vi "Main.vi"() -> ()   [LabVIEW 2024]
doc: "This template is for the Queued Message Handler design pattern.\n\nThe Event Handling Loop generates messages based on user interface actions.\n\nThe Message Handling Loop processes messages generated by the Event Handling Loop, or by other messages. The messages are string values, so new messages can be added easily to the Message Cases case structure in the Message Handling Loop. Each message cluster can also provide an optional value for Message Data, which is a variant that can be converted to whatever message-specific data is required."
uses:
  support/Message Queue/Enqueue Message (Single).vi
  <vilib>/Utility/error.llb/Error Cluster From Error Code.vi
  <vilib>/ErrorRing/Error Ring.xnode
  support/Message Queue/Message Queue.lvlib
  support/User Event - Stop/User Event - Stop.lvlib
panel:
  in  "Path":path
  out "Waveform Graph":dbl[](graph)
  out "Status":string
  in  "Open file":bool
  in  "Exit":bool
  # "File Reader lab 5"
  # "C:\\Users\\danfr\\Documents\\Studie\\V25\\FYS4240 - Datainnsamling og Kontroll\\Lab\\lab5_v25\\Example Binary File.dat"
  # "Path to the binary file on my computer"
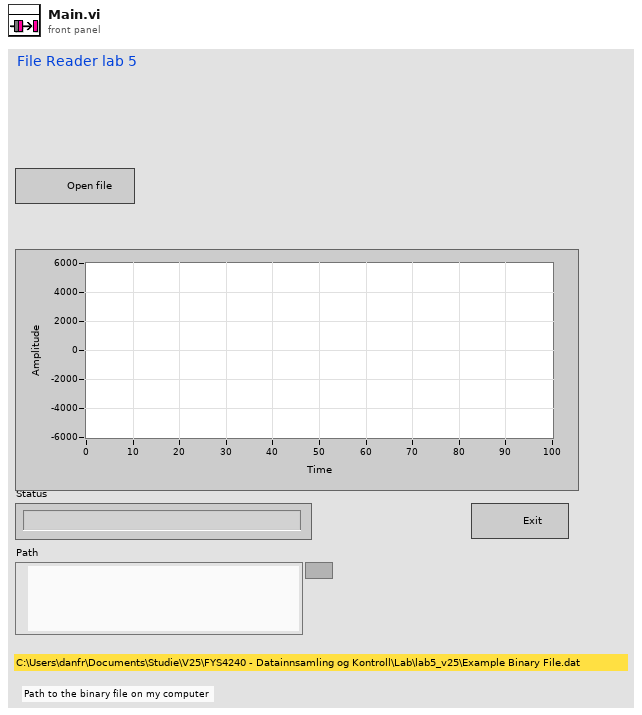
[diagram p1: front panel]
types:
  T1 = typedef "Message Queue.lvlib/All Message Queues.ctl" = cluster{"UI":refnum<queue>}
  T2 = enum16{"open", "replace", "create", "open or create", "replace or create", "replace or create with confirmation"}
  T3 = enum16{"big-endian, network order", "native, host order", "little-endian"}
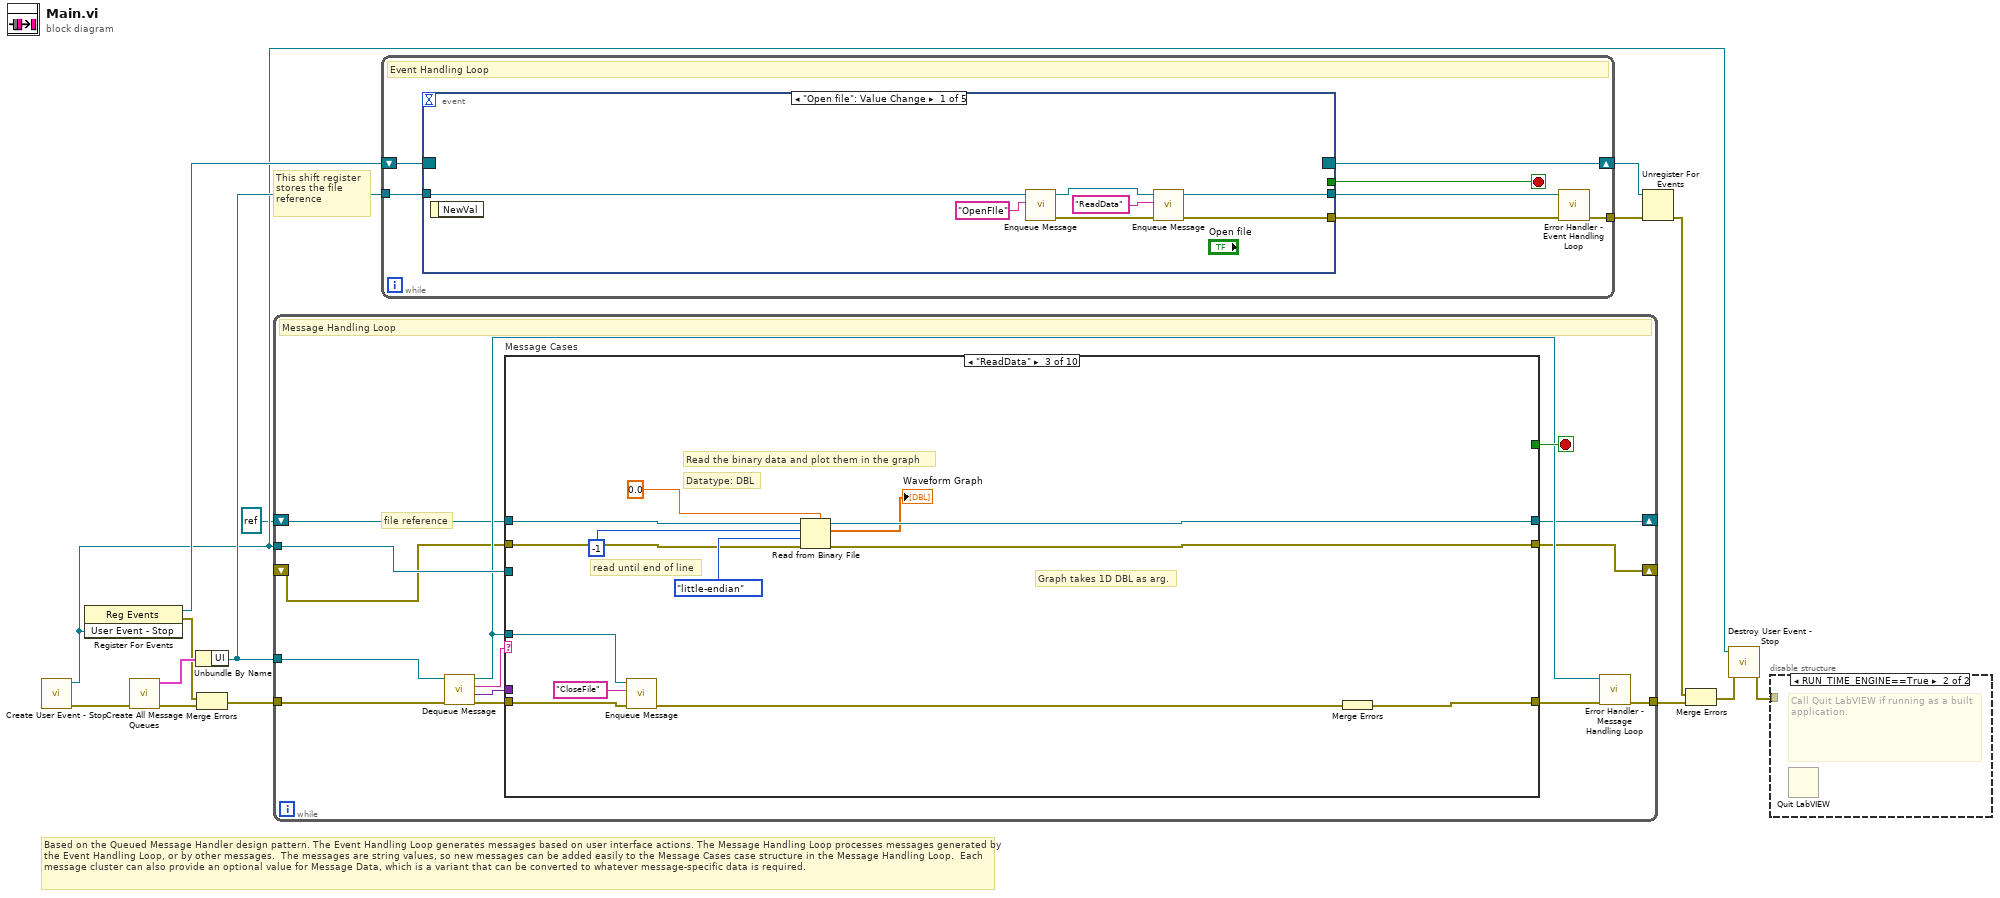
[diagram p0: block diagram]
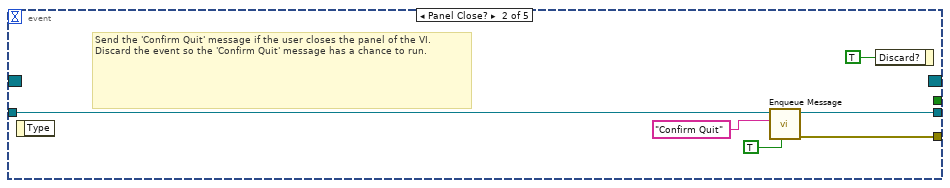
[diagram p3: hidden frame]
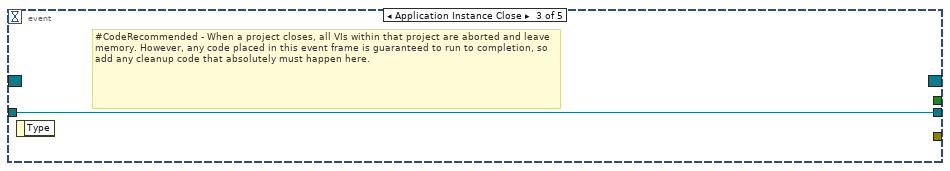
[diagram p4: hidden frame]
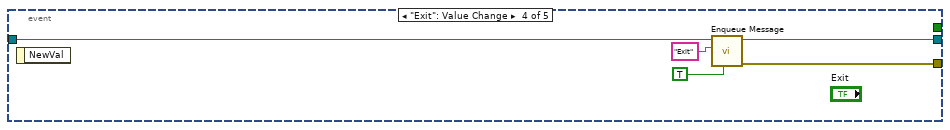
[diagram p5: hidden frame]
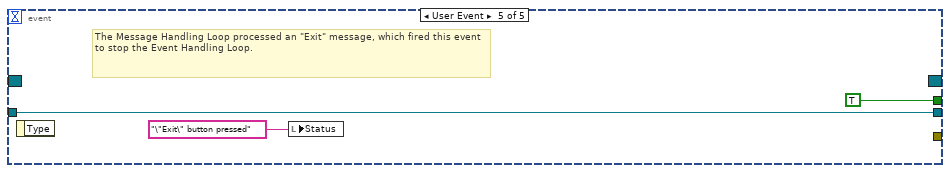
[diagram p6: hidden frame]
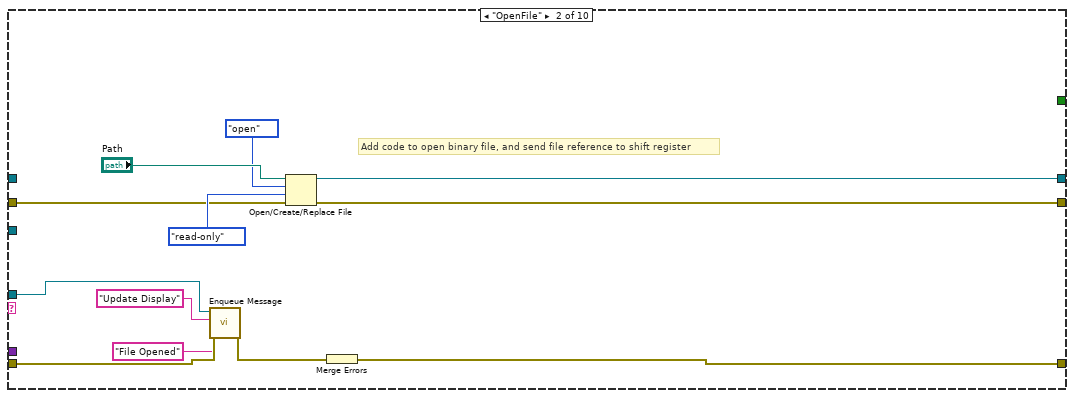
[diagram p8: hidden frame]
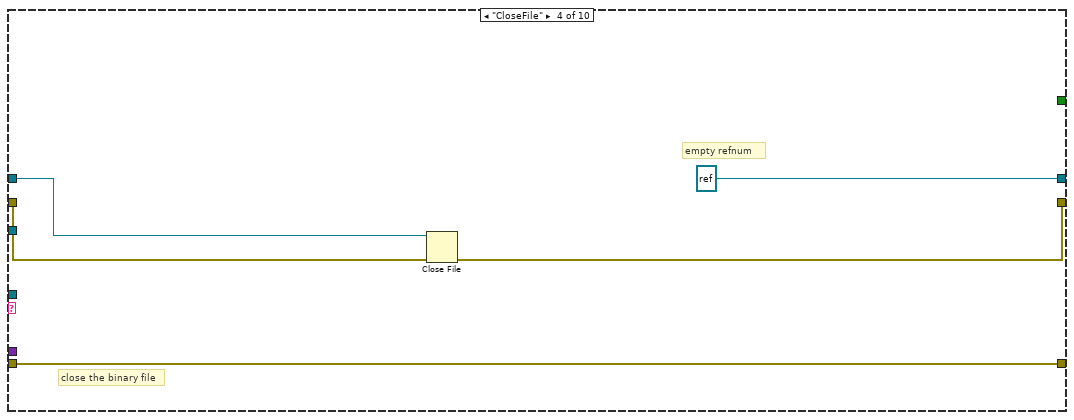
[diagram p9: hidden frame]
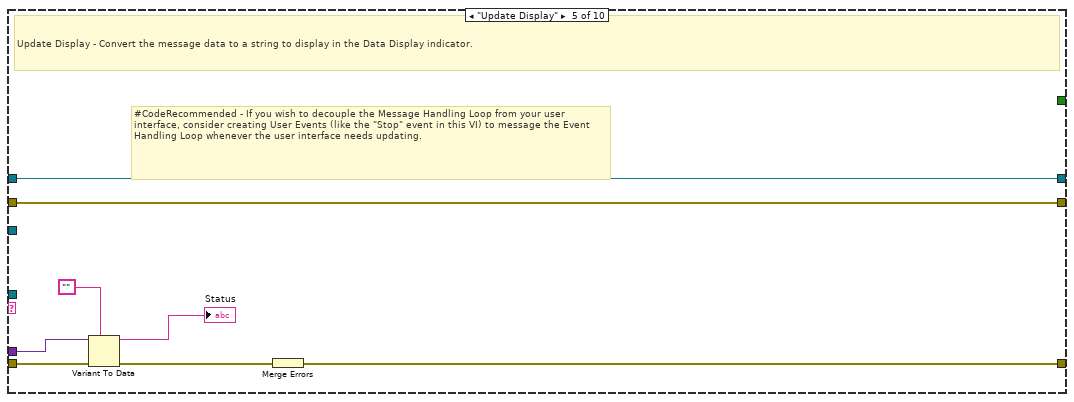
[diagram p10: hidden frame]
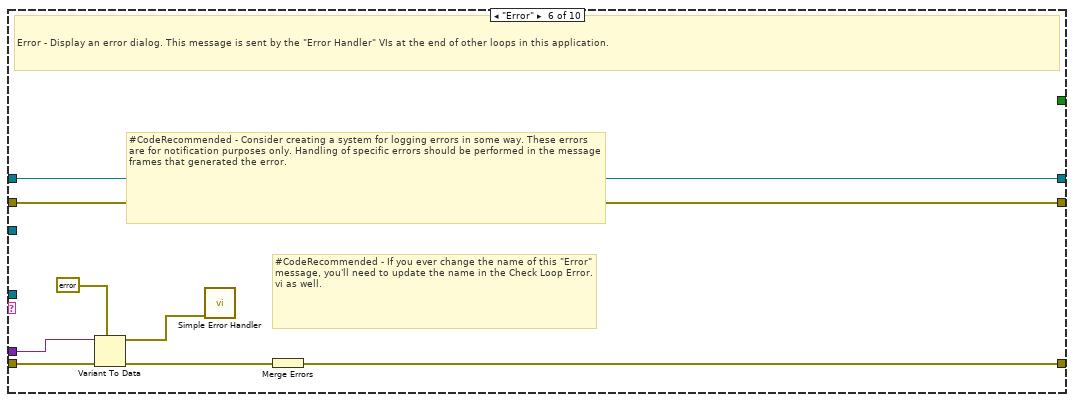
[diagram p11: hidden frame]
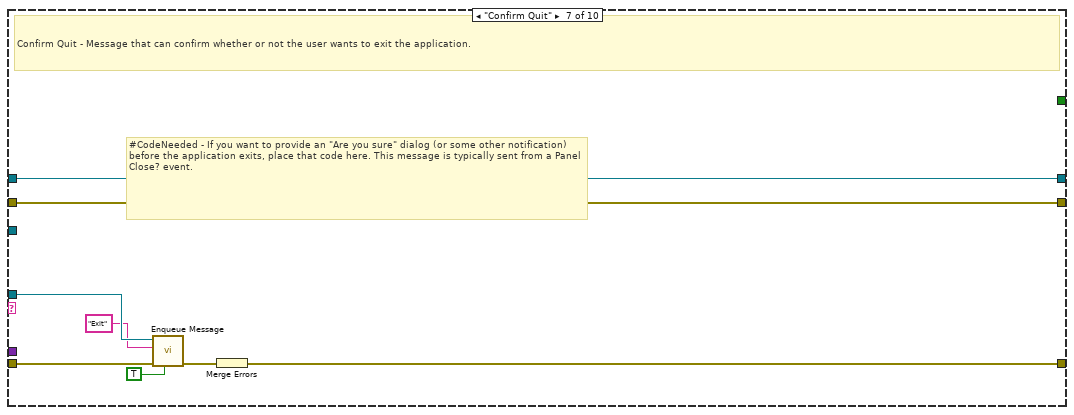
[diagram p12: hidden frame]
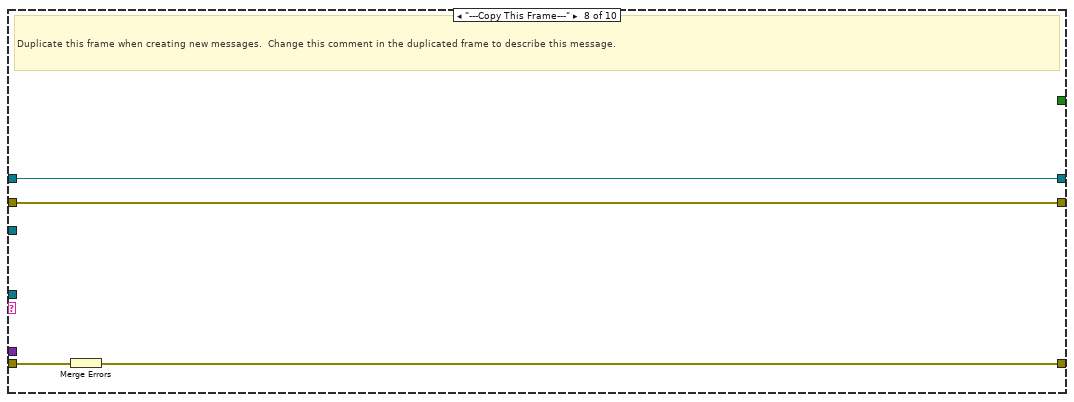
[diagram p13: hidden frame]
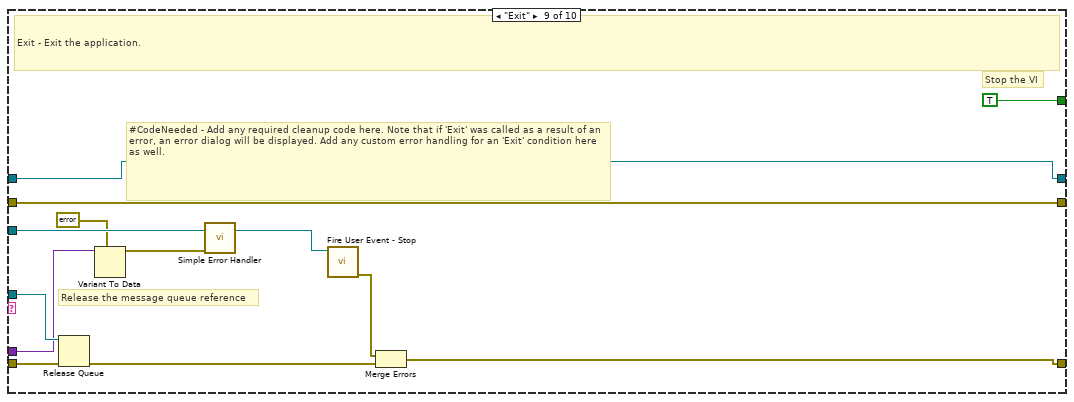
[diagram p14: hidden frame]
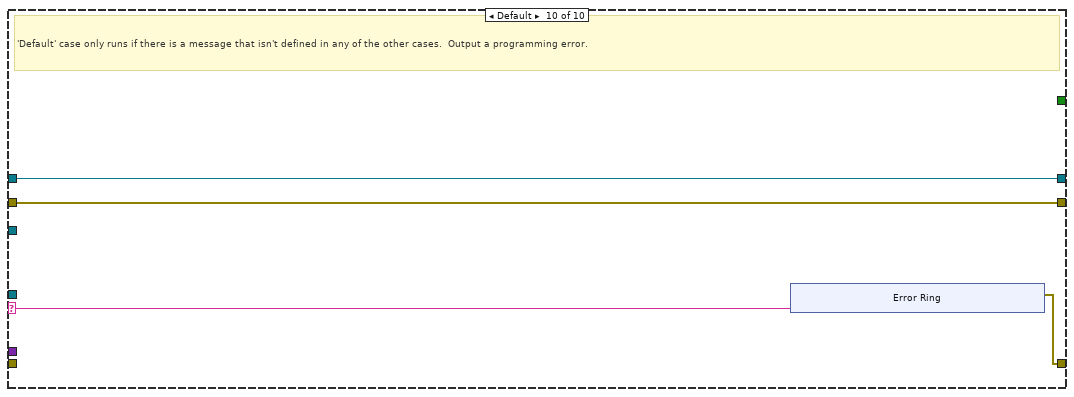
[diagram p15: hidden frame]
diagram:
  # "Based on the Queued Message Handler design pattern. The Event Handling Loop generates messages based on user interface actions. The Message Handling Loop processes messages generated by the Event Handling Loop, or by other messages.  The messages are string values, so new messages can be added easily to the Message Cases case structure in the Message Handling Loop.  Each message cluster can also provide an optional value for Message Data, which is a variant that can be converted to whatever message-specific data is required."
  # "This shift register stores the file reference"
  n1 = call "Create User Event - Stop.vi"() -> ("error out"=w11:errorcluster, "User Event - Stop"=w4:refnum<user-event>)  [unwired: 10 in]
  n2 = register-events(w4) -> (reference out=w5:refnum<event-registration>, error out=w2:errorcluster)  [unwired: 2 in]
  n3 = call "Create All Message Queues.vi"("error in (no error)"=w11) -> ("error out"=w15:errorcluster, "Message Queues out"=w14:T1)  [unwired: 9 in]
  n4 = Unbundle By Name(w14) -> ("UI"=w12:refnum<queue>)
  n5 = Merge Errors(w2, w15) -> (w3:errorcluster)
  n6 = while {
    tunnel: w12 -> [w23]
    tunnel: w4 -> [w28]
    tunnel: w3 -> [w27]
    tunnel: [w21] -> w13
    shift-right: [w18] -> _
    shift-left: refnum<file> refnum ("refnum out") -> [w19]
    shift-right: [w17] -> _
    shift-left: _ -> [w16]
    stop <- w29 stop-if-true
    # "file reference"
    # "Message Handling Loop"
    n7 = call "Dequeue Message.vi"("error in (no error)"=w27, "Message Queue"=w23) -> ("error out"=w26:errorcluster, "Message Data"=w24:variant, "Message"=w25:string, "dup Message Queue"=w22:refnum<queue>)  [unwired: 6 in]
    n8 = case "Message Cases" shown="\"ReadData\"" w25 {
      selector: w25 -> [_ _ _ _ _ _ _ _ _ w105]
      tunnel: w22 -> [_ w41 w54 _ _ _ w83 _ w102 _]
      tunnel: w26 -> [w32 w43 w56 w62 w69 w78 w86 w90 w96 _]
      tunnel: [w32 w44 w57 w62 w70 w73 w85 w89 w99 w106] -> w20
      tunnel: [_ _ _ _ _ _ _ _ TRUE _] -> w29
      tunnel: w24 -> [_ _ _ _ w68 w77 _ _ w93 _]
      tunnel: w28 -> [_ _ _ _ _ _ _ _ w98 _]
      tunnel: w19 -> [w31 _ w52 w61 w64 w72 w80 w88 w92 w104]
      tunnel: [w31 w36 w51 refnum<file> refnum ("refnum") w64 w72 w80 w88 w92 w104] -> w18
      tunnel: [w30 w33 w46 w59 w63 w71 w79 w87 w91 w103] -> w17
      tunnel: w16 -> [w30 w34 w45 w58 w63 w71 w79 w87 w91 w103]
      frame "Initialize" {
        # "Nothing added here in this example"
        # "Initialize - All initialization work should take place in this message, since other loops can potentially enqueue messages that execute immediately after this one."
      }
      frame "OpenFile" {
        # "Add code to open binary file, and send file reference to shift register"
        n9 = call-poly "Enqueue Message.vi"("error in (no error)"=w43, "Message Data"="File Opened" ("\"Do Something\" button pressed"), "Message"="Update Display", "Message Queue"=w41) -> ("error out"=w42:errorcluster)  [unwired: 6 in, 1 out]
        n10 = Open/Create/Replace File(file path (use dialog)="Path", error in=w34, operation (0:open)=T2."open", access (0:read/write)=enum16{"read/write", "read-only", "write-only"}."read-only") -> (refnum out=w36:refnum<file>, error out=w33:errorcluster)  [unwired: 2 in, 1 out]
        n11 = Merge Errors(w42) -> (w44:errorcluster)
      }
      frame "ReadData" {
        # "read until end of line"
        # "Graph takes 1D DBL as arg."
        # "Datatype: DBL"
        # "Read the binary data and plot them in the graph"
        n12 = call-poly "Enqueue Message.vi"("error in (no error)"=w56, "Message"="CloseFile", "Message Queue"=w54) -> ("error out"=w55:errorcluster)  [unwired: 7 in, 1 out]
        n13 = Read from Binary File(5:0.0, 8:w45, 9:T3."little-endian" ("byte order (0:big-endian, network order)"), 10:-1 ("count (1)"), 11:w52) -> (0:w46:errorcluster, 2:→"Waveform Graph":dbl[], 3:w51:refnum<file>)  [unwired: 1 in, 1 out]
        n14 = Merge Errors(w55) -> (w57:errorcluster)
      }
      frame "CloseFile" {
        # "empty refnum"
        # "close the binary file"
        n15 = Close File(refnum=w61, error in=w58) -> (error out=w59:errorcluster)  [unwired: 1 out]
      }
      frame "Update Display" {
        # "#CodeRecommended - If you wish to decouple the Message Handling Loop from your user interface, consider creating User Events (like the \"Stop\" event in this VI) to message the Event Handling Loop whenever the user interface needs updating."
        # "Update Display - Convert the message data to a string to display in the Data Display indicator."
        n16 = Variant To Data(error in=w69, type="", Variant=w68) -> (data=→"Status":string, error out=w66:errorcluster)
        n17 = Merge Errors(w66) -> (w70:errorcluster)
      }
      frame "Error" {
        # "#CodeRecommended - If you ever change the name of this \"Error\" message, you'll need to update the name in the Check Loop Error.vi as well."
        # "#CodeRecommended - Consider creating a system for logging errors in some way. These errors are for notification purposes only. Handling of specific errors should be performed in the message frames that generated the error."
        # "Error - Display an error dialog. This message is sent by the \"Error Handler\" VIs at the end of other loops in this application."
        n18 = Variant To Data(error in=w78, type=errorcluster {"status"=FALSE, "code"=0, "source"=""} ("error constant"), Variant=w77) -> (data=w75:errorcluster, error out=w74:errorcluster)
        n19 = call <vilib>:"Simple Error Handler.vi"("error in (no error)"=w75) -> ()  [unwired: 4 in, 5 out]
        n20 = Merge Errors(w74) -> (w73:errorcluster)
      }
      frame "Confirm Quit" {
        # "#CodeNeeded - If you want to provide an \"Are you sure\" dialog (or some other notification) before the application exits, place that code here. This message is typically sent from a Panel Close? event."
        # "Confirm Quit - Message that can confirm whether or not the user wants to exit the application."
        n21 = call-poly "Enqueue Message.vi"("Priority Message? (F)"=TRUE, "error in (no error)"=w86, "Message"="Exit", "Message Queue"=w83) -> ("error out"=w84:errorcluster)  [unwired: 6 in, 1 out]
        n22 = Merge Errors(w84) -> (w85:errorcluster)
      }
      frame "---Copy This Frame---" {
        # "Duplicate this frame when creating new messages.  Change this comment in the duplicated frame to describe this message."
        n23 = Merge Errors(w90) -> (w89:errorcluster)
      }
      frame "Exit" {
        # "Stop the VI"
        # "Release the message queue reference"
        # "#CodeNeeded - Add any required cleanup code here. Note that if 'Exit' was called as a result of an error, an error dialog will be displayed. Add any custom error handling for an 'Exit' condition here as well."
        # "Exit - Exit the application."
        n24 = Release Queue(queue=w102, error in (no error)=w96) -> (error out=w100:errorcluster)  [unwired: 1 in, 2 out]
        n25 = Variant To Data(type=errorcluster {"status"=FALSE, "code"=0, "source"=""} ("error constant"), Variant=w93) -> (data=w94:errorcluster)  [unwired: 1 in, 1 out]
        n26 = call <vilib>:"Simple Error Handler.vi"("error in (no error)"=w94) -> ()  [unwired: 4 in, 5 out]
        n27 = call "Fire User Event - Stop.vi"("User Event - Stop"=w98) -> ("error out"=w97:errorcluster)  [unwired: 10 in]
        n28 = Merge Errors(w97, w100) -> (w99:errorcluster)
      }
      frame Default {
        # "'Default' case only runs if there is a message that isn't defined in any of the other cases.  Output a programming error."
        n29 = xnode "Error Ring"("parameter 0"=w105) -> ("error out"=w106:errorcluster)
      }
    }
    n30 = call "Error Handler - Message Handling Loop.vi"("error in (no error)"=w20, "Message Queue"=w22) -> ("dup error in"=w21:errorcluster)  [unwired: 8 in, 1 out]
  }
  n31 = while {
    tunnel: w12 -> [w120]
    shift-right: [w118] -> w8
    shift-left: w5 -> [w119]
    tunnel: [w114] -> w6
    stop <- w116 stop-if-true
    # "Event Handling Loop"
    n32 = event shown="[0] \"Open file\": Value Change" {
      selector: w119 -> [_ _ _ _ _]
      dyn-events: [_ _ _ _ _] -> w118
      timeout: _ -> [_ _ _ _ _]
      tunnel: [_ _ _ _ TRUE ("Discard?")] -> w116
      tunnel: w120 -> [w127 w132 w134 w139 w142]
      tunnel: [w121 w131 _ w138 _] -> w117
      tunnel: [w122 w130 w134 w137 w142] -> w115
      event "Open file": Value Change {
        n33 = event-data() -> ()  [unwired: 1 in, 1 out]
        n34 = call-poly "Enqueue Message.vi"("Message"="OpenFIle", "Message Queue"=w127) -> ("error out"=w124:errorcluster, "dup Message Queue"=w125:refnum<queue>)  [unwired: 8 in]
        n35 = call-poly "Enqueue Message.vi"("error in (no error)"=w124, "Message"="ReadData", "Message Queue"=w125) -> ("error out"=w121:errorcluster, "dup Message Queue"=w122:refnum<queue>)  [unwired: 7 in]
      }
      event Panel Close? {
        # "Send the 'Confirm Quit' message if the user closes the panel of the VI. Discard the event so the 'Confirm Quit' message has a chance to run."
        n36 = event-data() -> ()  [unwired: 1 in, 1 out]
        n37 = call-poly "Enqueue Message.vi"("Priority Message? (F)"=TRUE, "Message"="Confirm Quit", "Message Queue"=w132) -> ("error out"=w131:errorcluster, "dup Message Queue"=w130:refnum<queue>)  [unwired: 7 in]
        n38 = event-data("Discard?"=TRUE) -> ()  [unwired: 1 in, 1 out]
      }
      event Application Instance Close {
        # "#CodeRecommended - When a project closes, all VIs within that project are aborted and leave memory. However, any code placed in this event frame is guaranteed to run to completion, so add any cleanup code that absolutely must happen here."
        n39 = event-data() -> ()  [unwired: 1 in, 1 out]
      }
      event "Exit": Value Change {
        n40 = event-data() -> ()  [unwired: 1 in, 1 out]
        n41 = call-poly "Enqueue Message.vi"("Priority Message? (F)"=TRUE, "Message"="Exit", "Message Queue"=w139) -> ("error out"=w138:errorcluster, "dup Message Queue"=w137:refnum<queue>)  [unwired: 7 in]
      }
      event User Event {
        # "The Message Handling Loop processed an \"Exit\" message, which fired this event to stop the Event Handling Loop."
        n42 = event-data() -> ()  [unwired: 1 in, 1 out]
        n43 = local write "Status"("\"Exit\" button pressed" ("VI Stopped")) -> ()
      }
    }
    n44 = call "Error Handler - Event Handling Loop.vi"("error in (no error)"=w117, "Message Queue"=w115) -> ("dup error in"=w114:errorcluster)  [unwired: 8 in, 1 out]
  }
  n45 = Unregister For Events(event registration refnum=w8, error in=w6) -> (error out=w9:errorcluster)
  n46 = Merge Errors(w9, w13) -> (w10:errorcluster)
  n47 = call "Destroy User Event - Stop.vi"("error in (no error)"=w10, "User Event - Stop"=w4) -> ("error out"=w7:errorcluster)  [unwired: 9 in]
  n48 = disable-structure shown="RUN_TIME_ENGINE==True" {
    disable-tunnel: w7 -> [_ _]
    frame condition #0 (active) {
    }
    frame condition #1 {
      # "Call Quit LabVIEW if running as a built application."
      n49 = Quit LabVIEW() -> ()  [unwired: 1 in]
    }
  }
